vi "WSVCAP SHL Host TL I2C Read.vi"(0 "Bytes to Read":u8=8, 5 "Sub Address [U8]":u8=191 format="%.0x", 7 "Socket Mask [U64]":u64=1 format="%016x", 11 "error in":errorcluster, 13 "Log (T)":bool=TRUE) -> (4 "C1 Read Data Out":u8[][](array[numeric]) format="%.0x", 6 "C2 Read Data Out":u8[][](array[numeric]) format="%.0x", 8 "C3 Read Data Out":u8[][](array[numeric]) format="%.0x", 15 "error out":errorcluster)   [LabVIEW 2012]
uses:
  Type Defs/WSVCAP SHL Function Enum.ctl
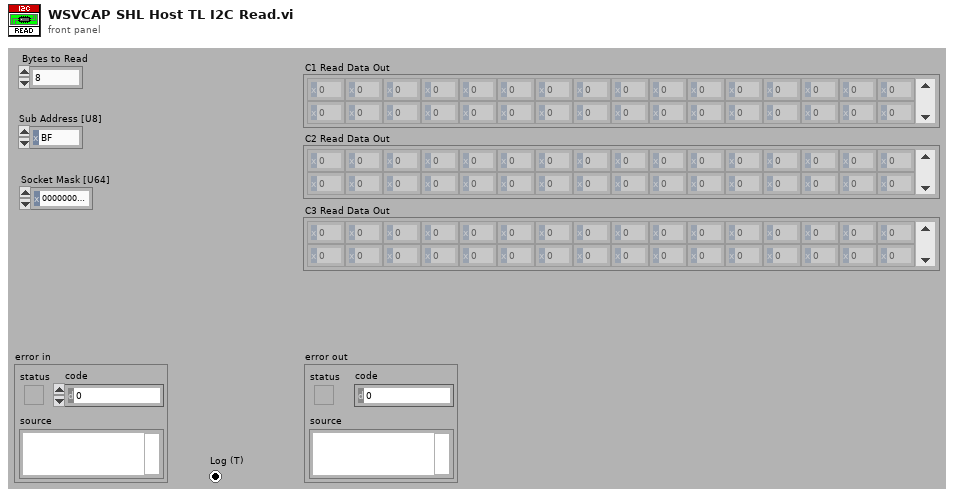
[diagram p1: front panel]
types:
  T1 = typedef "WSVCAP SHL Function Enum.ctl" = enum16{"Initialize", "Configure I2C", "Configure SPI", "Configure RFFE", "Write I2C", "Read I2C", "Write/Read SPI", "Start SPI Cycle", "Stop SPI Cycle", "Write RFFE", "Read RFFE", "Start RFFE Cycle", "Stop RFFE Cycle", "Get Status", "Close"}
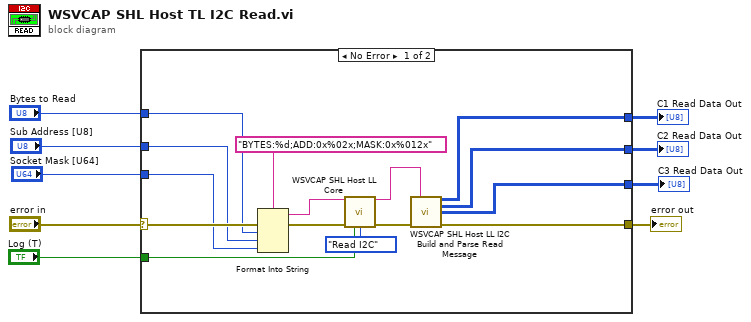
[diagram p0: block diagram]
diagram:
  n1 = case shown="No Error" "error in" {
    selector: "error in" -> [w19 w25]
    tunnel: [w23 w25] -> w8
    tunnel: [w21 _] -> w3
    tunnel: [w20 _] -> w2
    tunnel: "Bytes to Read" -> [w16 _]
    tunnel: "Sub Address [U8]" -> [w15 _]
    tunnel: "Socket Mask [U64]" -> [w14 _]
    tunnel: "Log (T)" -> [w11 _]
    tunnel: [w10 _] -> w1
    frame No Error {
      n2 = Format Into String(format string="BYTES:%d;ADD:0x%02x;MASK:0x%012x", error in=w19, w16, w15, w14) -> (resulting string=w13:string, error out=w18:errorcluster)  [unwired: 1 in]
      n3 = call "WSVCAP SHL Host LL Core.vi"("Message In"=w13, "error in"=w18, "Log (T)"=w11, "Function"=WSVCAP_SHL_Function_Enum."Read I2C") -> ("Message Out"=w22:string, "error out"=w24:errorcluster)  [unwired: 9 in, 1 out]
      n4 = call "WSVCAP SHL Host LL I2C Build and Parse Read Message.vi"("Message In"=w22, "error in"=w24) -> ("C1 Write Data Out"=w21:u8[][], "C2 Write Data Out"=w20:u8[][], "C3 Write Data Out"=w10:u8[][], "error out"=w23:errorcluster)  [unwired: 8 in, 2 out]
    }
    frame Error {
    }
  }
  "error out" <- w8
  "C3 Read Data Out" <- w1
  "C1 Read Data Out" <- w3
  "C2 Read Data Out" <- w2
